vi "MergeLockArrays.vi"(1 "Input Interlock Array In 1":T1[](array[typedef]), 2 "Input Interlock Array In 2":T1[](array[typedef])) -> (0 "Combined Interlock Array":T1[](array[typedef]))   [LabVIEW 2016]
uses:
  InterlockElement.ctl
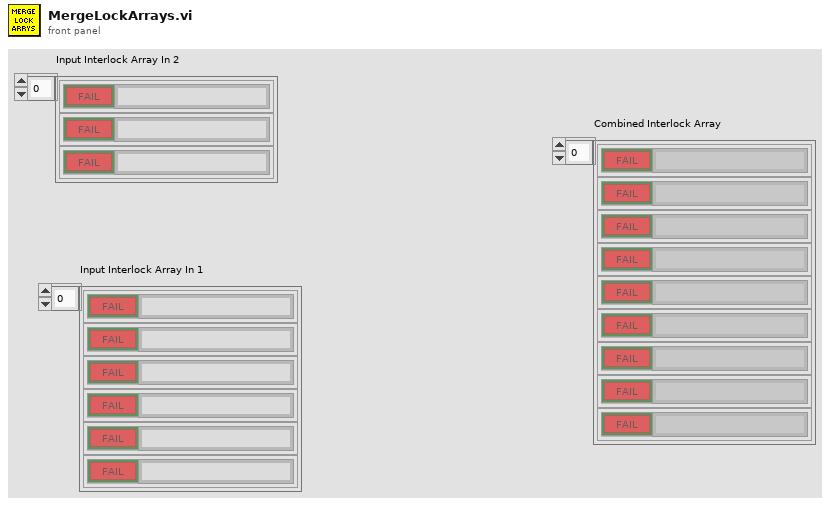
[diagram p1: front panel]
types:
  T1 = typedef "InterlockElement.ctl" = cluster{"Interlock State":bool, "Interlock Name":string}
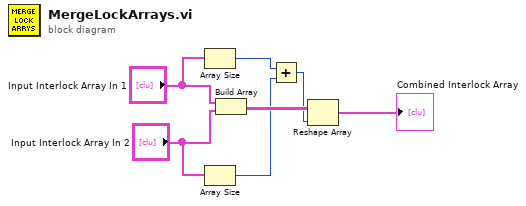
[diagram p0: block diagram]
diagram:
  n1 = Array Size(array="Input Interlock Array In 1") -> (size(s)=w3:i32)
  n2 = Array Size(array="Input Interlock Array In 2") -> (size(s)=w2:i32)
  n3 = Build Array("Input Interlock Array In 1", "Input Interlock Array In 2") -> (w7:T1[][])
  n4 = Add(x=w3, y=w2) -> (x+y=w1:i32)
  n5 = Reshape Array(w7, w1) -> (→"Combined Interlock Array":T1[])
